vi "rs3 release frame.vi"(8 "error in (no error)":errorcluster, 10 "Frame":u32, 11 "Device":u32) -> (0 "error out":errorcluster, 1 "error":u64, 3 "Device out":u32)   [LabVIEW 2017]
doc: "You MUST release the FRAME handle soon after you are done with it. It does not have to be immediately, but within about 15 frames."
uses:
  Users/Greg McKaskle/Downloads/librealsense-1.12.1/librealsense-1.12.1/bin/Win32/realsense-d.dll
panel:
  # "RS3 Release Frame"
  # "(C) Intel Corp. 2017,  AGJ"
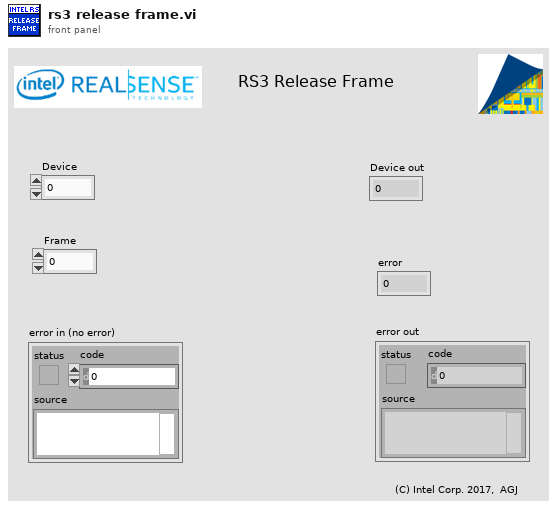
[diagram p1: front panel]
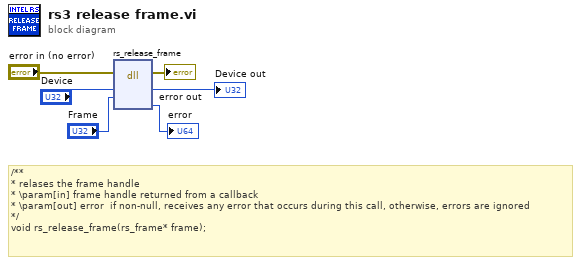
[diagram p0: block diagram]
diagram:
  # "/**\n* relases the frame handle\n* \\param[in] frame handle returned from a callback\n* \\param[out] error  if non-null, receives any error that occurs during this call, otherwise, errors are ignored\n*/\nvoid rs_release_frame(rs_frame* frame);"
  n1 = dll-call lib="C:/Users/Greg McKaskle/Downloads/librealsense-1.12.1/librealsense-1.12.1/bin/Win32/realsense-d.dll" fn="rs_release_frame"(error in="error in (no error)", "device"="Device", "frame"="Frame") -> (error out=→"error out":errorcluster, "device"=→"Device out":u64, "error"=→"error":u64)  [unwired: 5 in, 1 out]
